vi "Format Sum of Gaussians Fit Parameters.vi"(8 "Step Size":dbl, 9 "R^2":dbl, 10 "MSE":dbl, 11 "Best Fit Parameters":dbl[](array[numeric])) -> (0 "# Components":i32, 3 "Array of Gaussian Fit Parameters":T1[](array[typedef]))   [LabVIEW 2019]
uses:
  Gaussian/Gaussian Fit Results v2.ctl
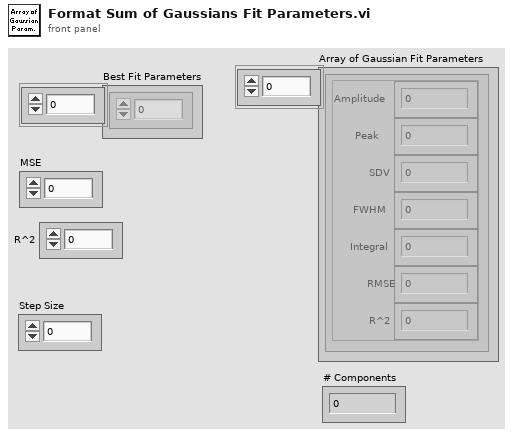
[diagram p1: front panel]
types:
  T1 = typedef "Gaussian Fit Results v2.ctl" = cluster{"Amplitude":dbl, "Peak":dbl, "SDV":dbl, "FWHM":dbl, "Integral":dbl, "RMSE":dbl, "R^2":dbl}
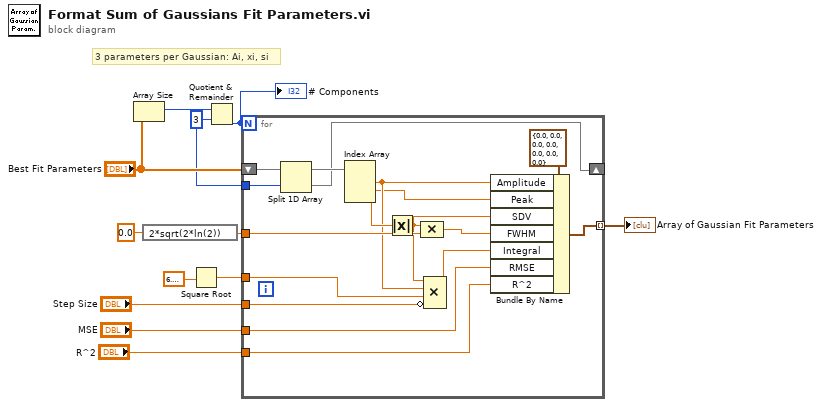
[diagram p0: block diagram]
diagram:
  w4 = 3 ("y")
  # "3 parameters per Gaussian: Ai, xi, si"
  n1 = Array Size(array="Best Fit Parameters") -> (size(s)=w6:i32)
  n2 = expression code="2*sqrt(2*ln(2))"(0.0) -> (w7:dbl)
  n3 = Square Root(x=6.283185307179586) -> (sqrt(x)=w9:dbl)
  n4 = Quotient & Remainder(x=w6, y=w4) -> (floor(x/y)=w2:i32)  [unwired: 1 out]
  "# Components" <- w2
  n5 = for {
    N: w2 -> [_]
    tunnel: w7 -> [w28]
    tunnel: w9 -> [w27]
    tunnel: "Step Size" -> [w26]
    tunnel: [w25] -> w10 mode=indexing
    tunnel: "MSE" -> [w14]
    shift-right: [w15] -> _
    shift-left: "Best Fit Parameters" -> [w18]
    tunnel: w4 -> [w17]
    tunnel: "R^2" -> [w13]
    n6 = Split 1D Array(array=w18, index=w17) -> (first subarray=w16:dbl[], second subarray=w15:dbl[])
    n7 = Index Array(array=w16) -> (element #1=w23:dbl, element #2=w22:dbl, element #3=w29:dbl)  [unwired: 3 in]
    n8 = Absolute Value(x=w29) -> (abs(x)=w21:dbl)
    n9 = Compound Arithmetic op=MULTIPLY(w21, w28) -> (w20:dbl)
    n10 = Compound Arithmetic op=MULTIPLY(w21, w23, w27, invert w26) -> (w19:dbl)
    n11 = Bundle By Name(cluster=T1 {"Amplitude"=0.0, "Peak"=0.0, "SDV"=0.0, "FWHM"=0.0, "Integral"=0.0, "RMSE"=0.0, "R^2"=0.0} ("Gaussian Fit Parameters"), "Amplitude"=w23, "Peak"=w22, "SDV"=w21, "FWHM"=w20, "Integral"=w19, "RMSE"=w14, "R^2"=w13) -> (w25:T1)
  }
  "Array of Gaussian Fit Parameters" <- w10
